vi "EXPRES Format Flipper Status Message.vi"(8 "error in":errorcluster, 10 "Mirrors":T1) -> (0 "error out":errorcluster, 2 "JSON string":string)   [LabVIEW 2016]
uses:
  Controls/Flip Mirrors.ctl
  Controls/Mirror Data.ctl
  Controls/Flip Mirror Status Message.ctl
  Controls/Messages/Mirror Message Struct.ctl
  Libs/Messages.lvlib
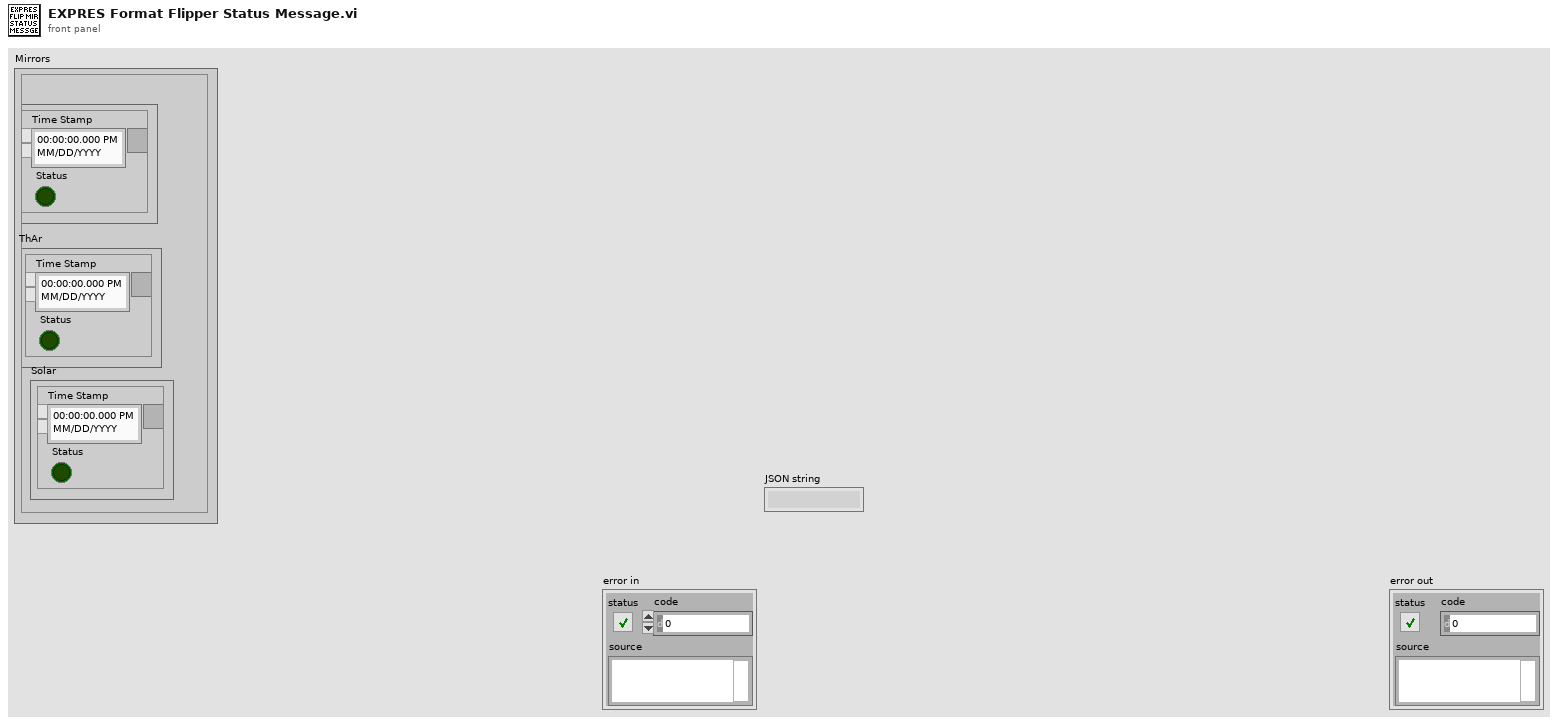
[diagram p1: front panel]
types:
  T1 = typedef "Flip Mirrors.ctl" = cluster{"ExtFlat":T2, "ThAr":T2, "Solar":T2}
  T2 = typedef "Mirror Data.ctl" = cluster{"Status":bool, "Time Stamp":timestamp}
  T3 = typedef "Messages.lvlib/Flip Mirror Status Message.ctl" = cluster{"ThAr":T4, "Ext Flat":T4, "Solar":T4}
  T4 = typedef "Messages.lvlib/Mirror Message Struct.ctl" = cluster{"status":string, "time":string}
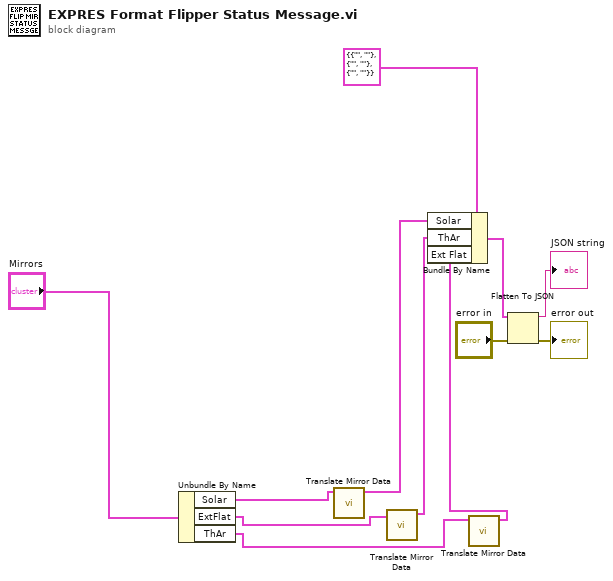
[diagram p0: block diagram]
diagram:
  n1 = Unbundle By Name("Mirrors") -> ("Solar"=w6:T2, "ExtFlat"=w4:T2, "ThAr"=w3:T2)
  n2 = call "Translate Mirror Data.vi"("Mirror"=w6) -> ("Mirror String"=w5:T4)  [unwired: 10 in]
  n3 = call "Translate Mirror Data.vi"("Mirror"=w4) -> ("Mirror String"=w2:T4)  [unwired: 10 in]
  n4 = call "Translate Mirror Data.vi"("Mirror"=w3) -> ("Mirror String"=w1:T4)  [unwired: 10 in]
  n5 = Bundle By Name(cluster=T3 {"ThAr"={"status"="", "time"=""}, "Ext Flat"={"status"="", "time"=""}, "Solar"={"status"="", "time"=""}}, "Solar"=w5, "ThAr"=w2, "Ext Flat"=w1) -> (w8:T3)
  n6 = Flatten To JSON(anything=w8, error in (no error)="error in") -> (JSON string=→"JSON string":string, 11:→"error out":errorcluster)  [unwired: 1 in]
